vi "Update Graphs 1D U16.vi"(8 "error in (no error)":errorcluster, 10 "image":u16[](array[numeric]), 11 "Detail Graph in":refnum<class "Detail Graph.lvclass">) -> (0 "error out":errorcluster, 1 "Cursor.Cursor Position":T1, 3 "Detail Graph out":refnum<class "Detail Graph.lvclass">)   [LabVIEW 2023, in "Detail Graph.lvclass"]
uses:
  Detail Graph.lvclass
  D:/git/Graph-Classes/source/Base Graph/Base Graph.lvclass
  <vilib>/Utility/miscctls.llb/LVPointDoubleTypeDef.ctl
  Base Graph/Base Graph.lvclass/Base Graph.ctl
  Detail Graph.lvclass/Detail Graph.ctl
  Base Graph/Base Graph.lvclass
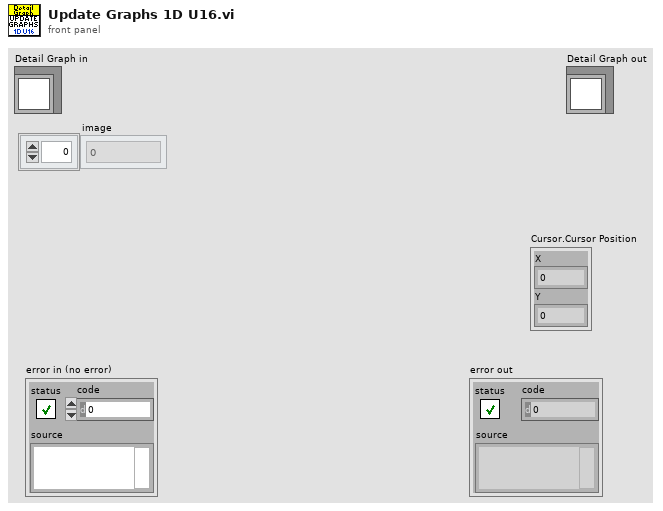
[diagram p1: front panel]
types:
  T1 = typedef "LVPointDoubleTypeDef.ctl" = cluster{"X":dbl, "Y":dbl}
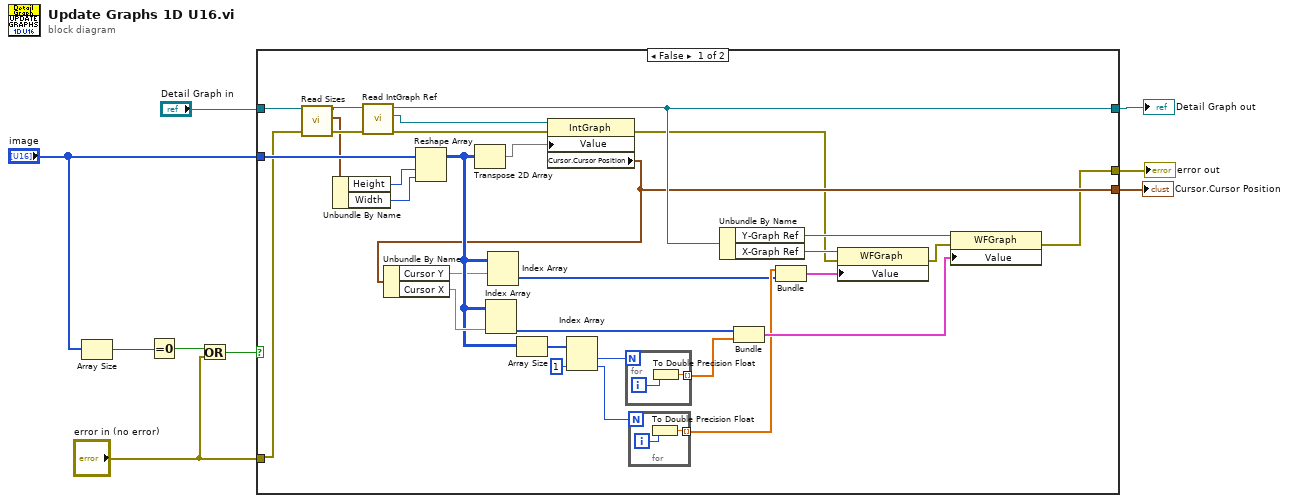
[diagram p0: block diagram]
diagram:
  n1 = Array Size(array="image") -> (size(s)=w1:i32)
  n2 = Equal To 0?(x=w1) -> (x = 0?=w6:bool)
  n3 = Or(x=w6, y="error in (no error)") -> (x .or. y?=w7:bool)
  n4 = case shown="False" w7 {
    tunnel: [w12 w44] -> w9
    tunnel: [w17 w45] -> w3
    tunnel: "Detail Graph in" -> [w22 w45]
    tunnel: "image" -> [w31 _]
    tunnel: "error in (no error)" -> [w23 w44]
    tunnel: [w14 _] -> w2
    frame False {
      n5 = call "Read Sizes.vi"("TG Base Graph in"=w22) -> ("Sizes"=w20:cluster{"Height":u32, "Width":u32}, "TG Base Graph out"=w21:refnum<class "Detail Graph.lvclass">)  [unwired: 8 in, 1 out]
      n6 = Unbundle By Name(w20) -> ("Height"=w18:u32, "Width"=w10:u32)
      n7 = call "Read IntGraph Ref.vi"("error in (no error)"=w23, "TG Base Graph in"=w21) -> ("error out"=w16:errorcluster, "IntGraph Ref"=w15:refnum<vi>, "TG Base Graph out"=w17:refnum<class "Detail Graph.lvclass">)  [unwired: 7 in]
      n8 = Reshape Array(w31, w18, w10) -> (w19:u16[][])
      n9 = Transpose 2D Array(2D array=w19) -> (transposed array=w37:u16[][])
      n10 = Array Size(array=w19) -> (size(s)=w39:i32[])
      n11 = property class="IntGraph"(reference=w15, error in=w16, "Value"=w37) -> (error out=w13:errorcluster, "Cursor.Cursor Position"=w14:T1)  [unwired: 1 out]
      n12 = Unbundle By Name(w14) -> ("Cursor Y"=w11:dbl, "Cursor X"=w34:dbl)
      n13 = Index Array(array=w19, index (col)=w34) -> (element=w32:u16[])  [unwired: 1 in]
      n14 = Index Array(array=w19, index (row)=w11) -> (element=w24:u16[])  [unwired: 1 in]
      n15 = Index Array(array=w39, index #2=1 ("index")) -> (element #1=w38:i32, element #2=w35:i32)  [unwired: 1 in]
      n16 = for {
        N: w38 -> [_]
        tunnel: [w43] -> w33 mode=indexing
        i -> [w42]
        n17 = To Double Precision Float(number=w42) -> (double precision float=w43:dbl)
      }
      n18 = for {
        N: w35 -> [_]
        tunnel: [w40] -> w25 mode=indexing
        i -> [w41]
        n19 = To Double Precision Float(number=w41) -> (double precision float=w40:dbl)
      }
      n20 = Unbundle By Name(w17) -> ("Y-Graph Ref"=w30:refnum<vi>, "X-Graph Ref"=w28:refnum<vi>)
      n21 = Bundle("image"=w32, w33) -> (w26:cluster{"image":u16[], dbl[]})  [unwired: 1 in]
      n22 = Bundle(w25, "image"=w24) -> (w27:cluster{dbl[], "image":u16[]})  [unwired: 1 in]
      n23 = property class="WFGraph"(reference=w28, error in=w13, "Value"=w27) -> (error out=w29:errorcluster)  [unwired: 1 out]
      n24 = property class="WFGraph"(reference=w30, error in=w29, "Value"=w26) -> (error out=w12:errorcluster)  [unwired: 1 out]
    }
    frame True {
    }
  }
  "error out" <- w9
  "Detail Graph out" <- w3
  "Cursor.Cursor Position" <- w2
